vi "Measure.vi"(7 "Num Iterations":i32, 8 "error in (no error)":errorcluster, 9 "Blow Out?":bool, 10 "Next Step":dbl[](array[numeric]), 11 "BaseProducer in":refnum<class "BaseProducer.lvclass">) -> (0 "error out":errorcluster, 1 "Blow Out?":bool, 2 "Temperature Array (C)":dbl[](array[numeric]), 3 "BaseProducer out":refnum<class "BaseProducer.lvclass">)   [LabVIEW 2013, in "BaseProducer.lvclass"]
doc: "This private method takes readings from sensors, checks for a flame, and returns some status. It needs to be given a number of iterations over which to proceed."
uses:
  BaseProducer.lvclass
  BaseProducer.lvclass/BaseProducer.ctl
  DbMeasurement/DbMeasurement.lvclass/DbMeasurement.ctl
  <vilib>/DAQmx/write.llb/DAQmx Write (Analog 1D DBL NChan 1Samp).vi
  <vilib>/DAQmx/read.llb/DAQmx Read (Analog 2D DBL NChan NSamp).vi
  <vilib>/DAQmx/read.llb/DAQmx Read (Analog 1D DBL NChan 1Samp).vi
  <vilib>/DAQmx/miscellaneous.llb/DAQmx Fill In Error Info.vi
  DbMeasurement/DbMeasurement.lvclass
panel:
  in  "Skip Button":bool
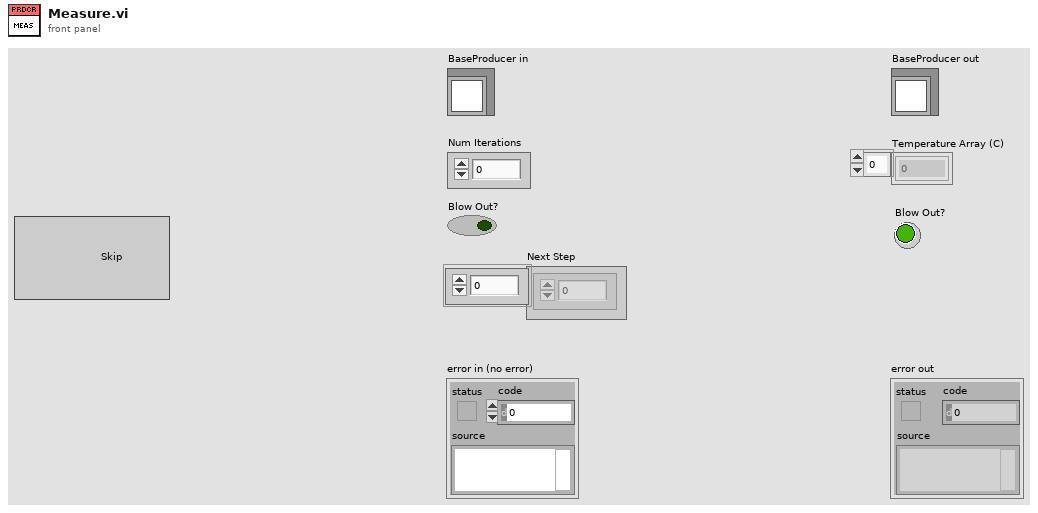
[diagram p1: front panel]
types:
  T1 = cluster{"P ATM":dbl, "JSON string":string, "JSON string":string, i16, "date/time string":string, "Waveform":dbl, "JSON string":string, "JSON string":string}
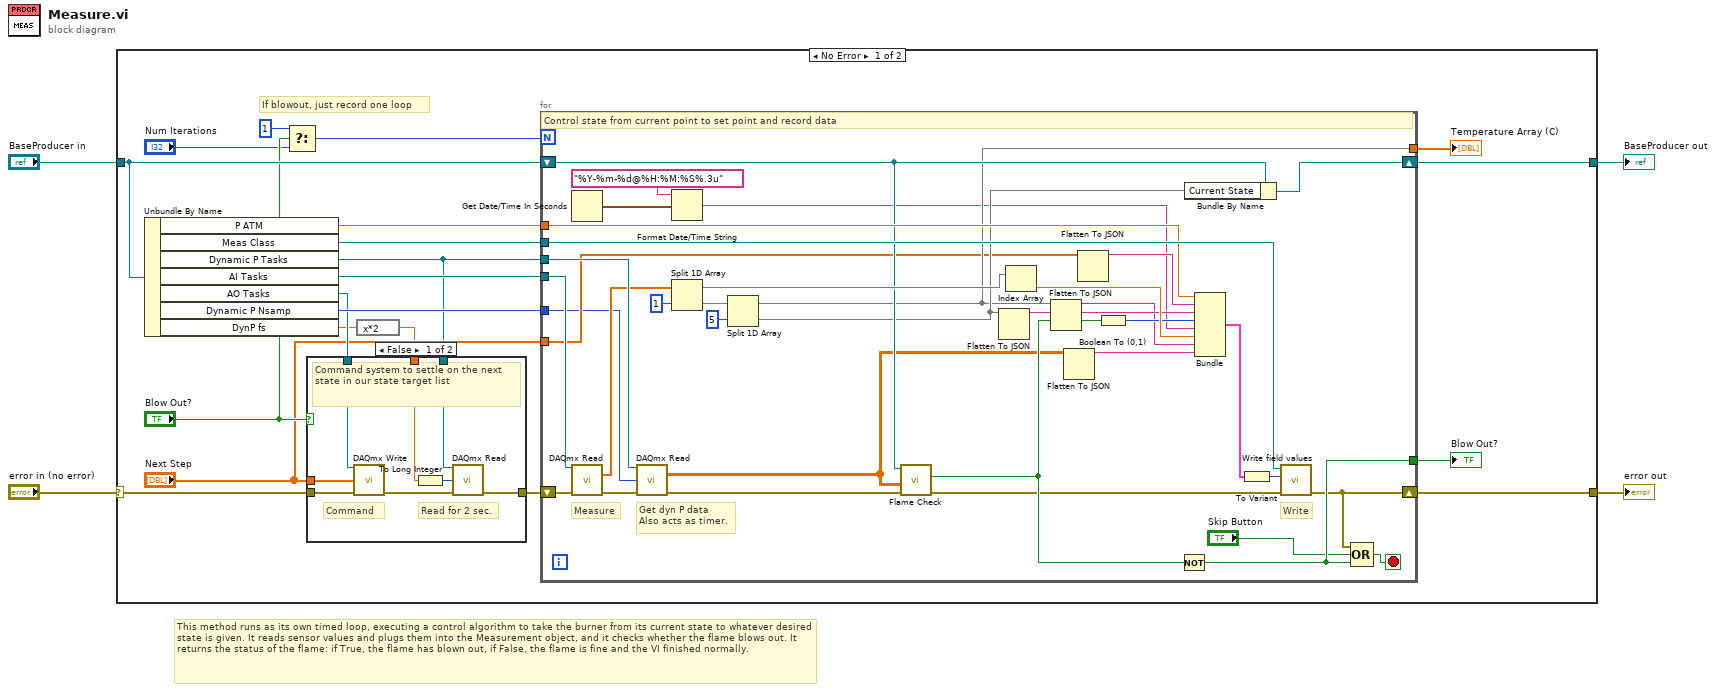
[diagram p0: block diagram]
diagram:
  # "This method runs as its own timed loop, executing a control algorithm to take the burner from its current state to whatever desired state is given. It reads sensor values and plugs them into the Measurement object, and it checks whether the flame blows out. It returns the status of the flame: if True, the flame has blown out, if False, the flame is fine and the VI finished normally."
  n1 = case shown="No Error" "error in (no error)" {
    selector: "error in (no error)" -> [w16 w71]
    tunnel: [w24 w71] -> w3
    tunnel: [w19 w70] -> w1
    tunnel: "BaseProducer in" -> [w20 w70]
    frame No Error {
      # "If blowout, just record one loop"
      n2 = Unbundle By Name(w20) -> ("P ATM"=w9:dbl, "Meas Class"=w23:refnum<class "DbMeasurement.lvclass">, "Dynamic P Tasks"=w7:refnum<k21>, "AI Tasks"=w22:refnum<k21>, "AO Tasks"=w15:refnum<k21>, "Dynamic P Nsamp"=w21:i32, "DynP fs"=w6:dbl)
      n3 = Select(t=1, s="Blow Out?", f="Num Iterations") -> (s? t:f=w11:i32)
      n4 = expression code="x*2"(w6) -> (w5:dbl)
      n5 = case shown="False" "Blow Out?" {
        tunnel: w16 -> [w32 w33]
        tunnel: w15 -> [w31 _]
        tunnel: [w28 w33] -> w14
        tunnel: "Next Step" -> [w30 _]
        tunnel: w7 -> [w27 _]
        tunnel: w5 -> [w26 _]
        frame False {
          # "Read for 2 sec."
          # "Command"
          # "Command system to settle on the next state in our state target list"
          n6 = call-poly <vilib>:"DAQmx Write.vi"("task/channels in"=w31, "data"=w30, "error in"=w32) -> ("error out"=w29:errorcluster)  [unwired: 10 in, 2 out]
          n7 = To Long Integer(number=w26) -> (32bit integer=w25:i32)
          n8 = call-poly <vilib>:"DAQmx Read.vi"("task/channels in"=w27, "number of samples per channel"=w25, "error in"=w29) -> ("error out"=w28:errorcluster)  [unwired: 10 in, 2 out]
        }
        frame True {
          # "Do not go to next. Used when we have a blowout and need to record it."
        }
      }
      n9 = for {
        N: w11 -> [_]
        shift-right: [w50] -> w24
        shift-left: w14 -> [w34]
        tunnel: w23 -> [w69]
        tunnel: w7 -> [w66]
        tunnel: w22 -> [w68]
        tunnel: w9 -> [w59]
        tunnel: [w41] -> w17
        shift-right: [w49] -> w19
        shift-left: w20 -> [w53]
        tunnel: [w54] -> w18
        tunnel: w21 -> [w35]
        tunnel: "Next Step" -> [w36]
        stop <- w52 stop-if-true
        # "Get dyn P data\nAlso acts as timer."
        # "Write"
        # "Measure"
        # "Control state from current point to set point and record data"
        n10 = Get Date/Time In Seconds() -> (seconds since 1Jan1904=w39:timestamp)
        n11 = call-poly <vilib>:"DAQmx Read.vi"("task/channels in"=w68, "error in"=w34) -> ("data"=w65:dbl[], "error out"=w67:errorcluster)  [unwired: 11 in, 1 out]
        n12 = call-poly <vilib>:"DAQmx Read.vi"("task/channels in"=w66, "number of samples per channel"=w35, "error in"=w67) -> ("data"=w47:dbl[][], "error out"=w58:errorcluster)  [unwired: 10 in, 1 out]
        n13 = Format Date/Time String(time format string (%c)="%Y-%m-%d@%H:%M:%S%.3u", seconds (now)=w39) -> (date/time string=w38:string)  [unwired: 1 in]
        n14 = Split 1D Array(array=w65, index=1) -> (first subarray=w56:dbl[], second subarray=w63:dbl[])
        n15 = Split 1D Array(array=w63, index=5) -> (first subarray=w41:dbl[], second subarray=w43:dbl[])
        n16 = call "Flame Check.vi"("error in (no error)"=w58, "Dynamic P data"=w47, "BaseProducer in"=w53) -> ("error out"=w45:errorcluster, "Flame?"=w57:bool)  [unwired: 6 in, 1 out]
        n17 = Flatten To JSON(anything=w43) -> (JSON string=w42:string)  [unwired: 2 in, 1 out]
        n18 = Index Array(array=w56) -> (element=w55:dbl)  [unwired: 1 in]
        n19 = Flatten To JSON(anything=w41) -> (JSON string=w40:string)  [unwired: 2 in, 1 out]
        n20 = Flatten To JSON(anything=w47) -> (JSON string=w46:string)  [unwired: 2 in, 1 out]
        n21 = Flatten To JSON(anything=w36) -> (JSON string=w44:string)  [unwired: 2 in, 1 out]
        n22 = Boolean To (0,1)(Boolean=w57) -> (0, 1=w48:i16)
        n23 = Not(x=w57) -> (.not. x?=w54:bool)
        n24 = Bundle By Name(cluster=w53, "Current State"=w43) -> (w49:refnum<class "BaseProducer.lvclass">)
        n25 = Bundle("P ATM"=w59, "JSON string"=w44, "JSON string"=w42, w48, "date/time string"=w38, "Waveform"=w55, "JSON string"=w40, "JSON string"=w46) -> (w62:T1)  [unwired: 1 in]
        n26 = To Variant(anything=w62) -> (Variant=w61:variant)
        n27 = call "Write field values.vi"("error in (no error)"=w45, "field values"=w61, "DbMeasurement in"=w69) -> ("error out"=w50:errorcluster)  [unwired: 7 in, 1 out]
        n28 = Compound Arithmetic op=OR(w50, "Skip Button", w54) -> (w52:bool)
      }
      "Blow Out?" <- w18
      "Temperature Array (C)" <- w17
    }
    frame Error {
    }
  }
  "error out" <- w3
  "BaseProducer out" <- w1
